vi "简易流程调试界面.vi"() -> ()   [LabVIEW 2016, in "斯坦道通用流路CODmn.lvlib"]
uses:
  <vilib>/Utility/miscctls.llb/LVPointTypeDef.ctl
  <vilib>/Plasmionique/MB Master/MB_Master/MB_Master.lvclass
panel:
  in  "调试控件":enum32{"填充流程", "清洗流程", "测试流程", "排空流程", "其他流程"}(tab)
  in  "填充简易流程":i32(listbox)
  in  "清洗简易流程":i32(listbox)
  in  "测试简易流程":i32(listbox)
  in  "排空简易流程":i32(listbox)
  in  "其他简易流程":i32(listbox)
  in  "停止":bool
  in  "单步测试":bool
  out "注射器温度":sgl
  out "消解温度":sgl
  out "ADC":sgl
  out "F3":sgl format="%#.6f"
  out "F2":sgl format="%#.6f"
  out "F1":sgl format="%#.6f"
  out "F0":sgl format="%#.6f"
  in  "启动":bool
  in  "参数下拉列表":u16(ring) items=["总磷"=1]
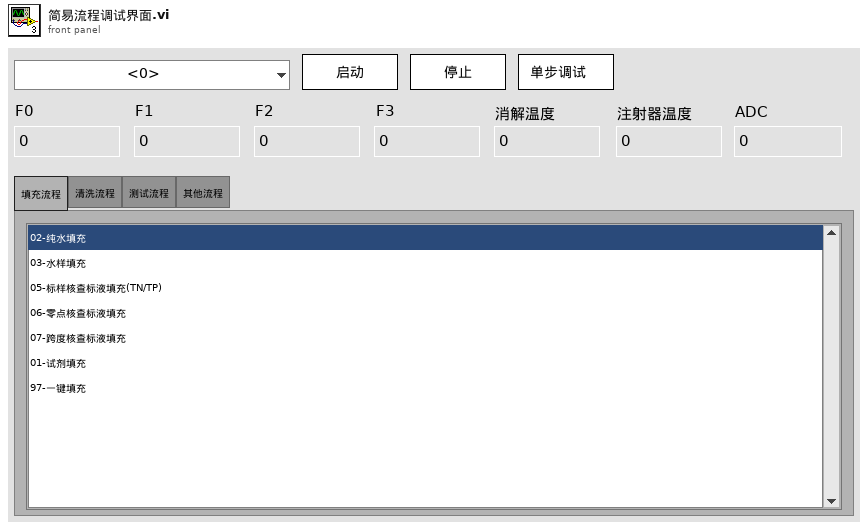
[diagram p1: front panel]
types:
  T1 = typedef "LVPointTypeDef.ctl" = cluster{"Horizontal":i16, "Vertical":i16}
  T2 = typedef "LVRectTypeDef.ctl" = cluster{"Left":i16, "Top":i16, "Right":i16, "Bottom":i16}
  T3 = typedef "LVStringsAndValuesArrayTypeDef_U16.ctl" = cluster{"String":string, "Value":u16}[]
  T4 = typedef "操作日志字段定义.ctl" = cluster{"时间":timestamp, "参数":string, "日志信息":string, "流程参数":string}
  T5 = enum16{"跨度核查", "水样测量", "零点核查", "标样核查", "加标回收", "快捷测试", "空白校准", "标样校准"}
  T6 = cluster{"系统时间":timestamp, "工作状态":u16, "测量模式":enum16{"待机", "连续模式", "周期模式", "定点模式", "受控模式", "手动模式"}, "告警代码":u16, "故障代码":u16, "日志代码":u16, "软件版本":u16, "F0":sgl, "F1":sgl, "F2":sgl, "F3":sgl, "T":sgl, "H":sgl, "id":u16, "flowid":u16, "量程":u16, "总磷控温温度1":sgl, "营养盐控温温度2":sgl, "ADC":sgl}
  T7 = enum32{"Bad", "Idle", "Run top level", "Running"}
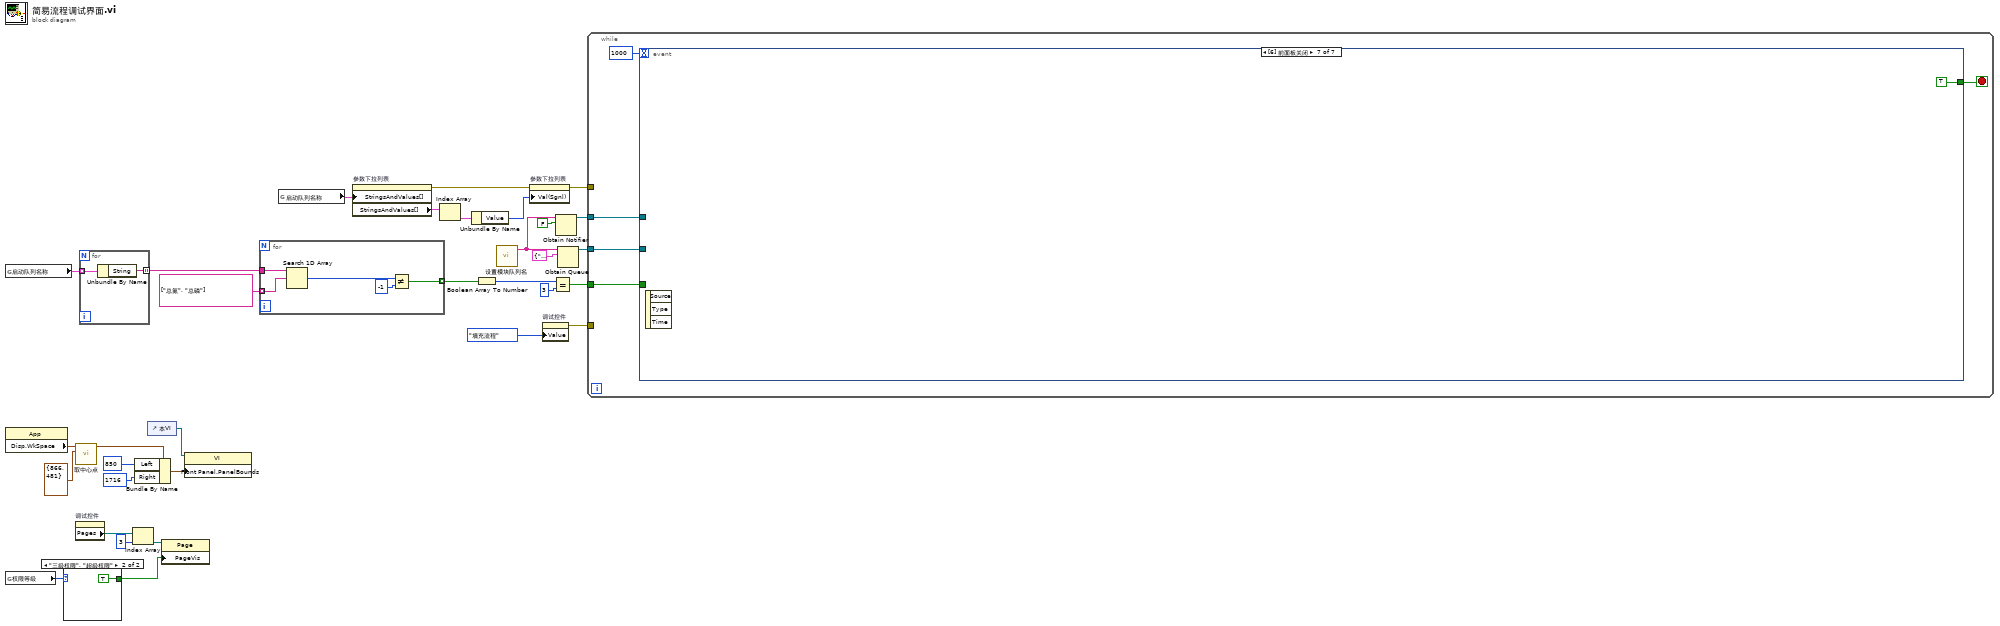
[diagram p0: block diagram]
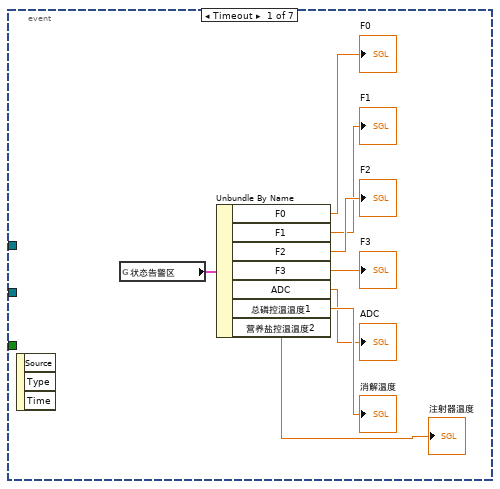
[diagram p3: hidden frame]
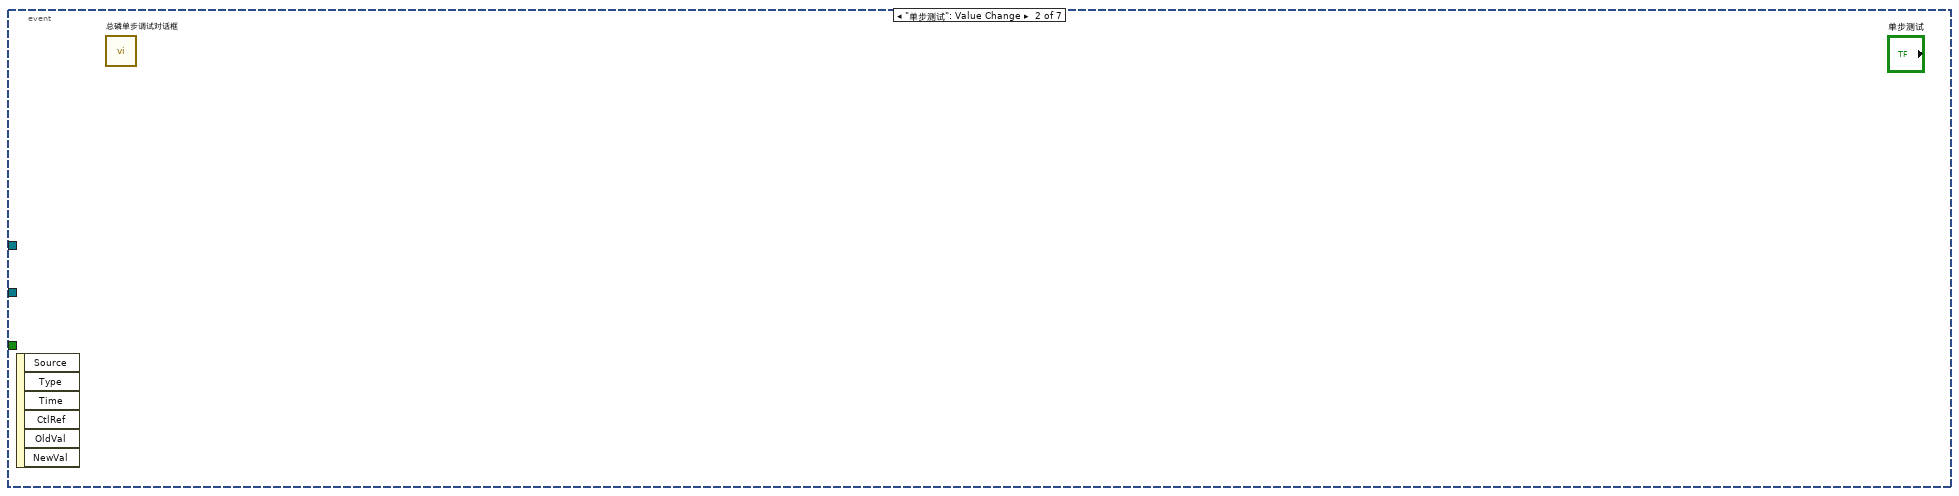
[diagram p4: hidden frame]
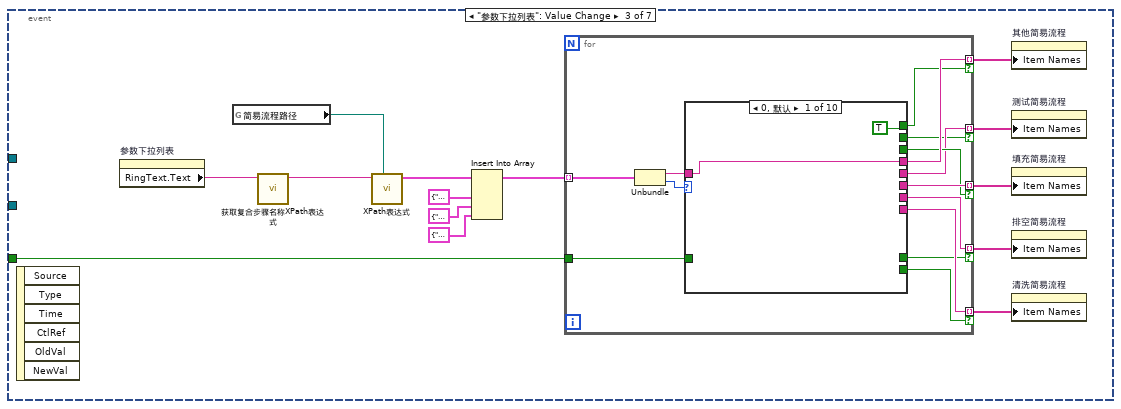
[diagram p5: hidden frame]
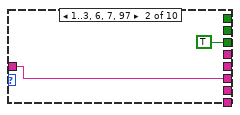
[diagram p6: hidden frame]
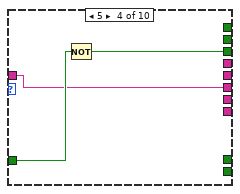
[diagram p8: hidden frame]
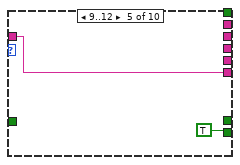
[diagram p9: hidden frame]
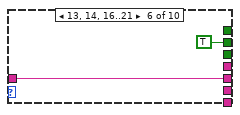
[diagram p10: hidden frame]
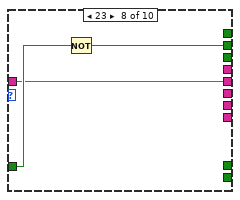
[diagram p12: hidden frame]
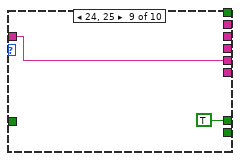
[diagram p13: hidden frame]
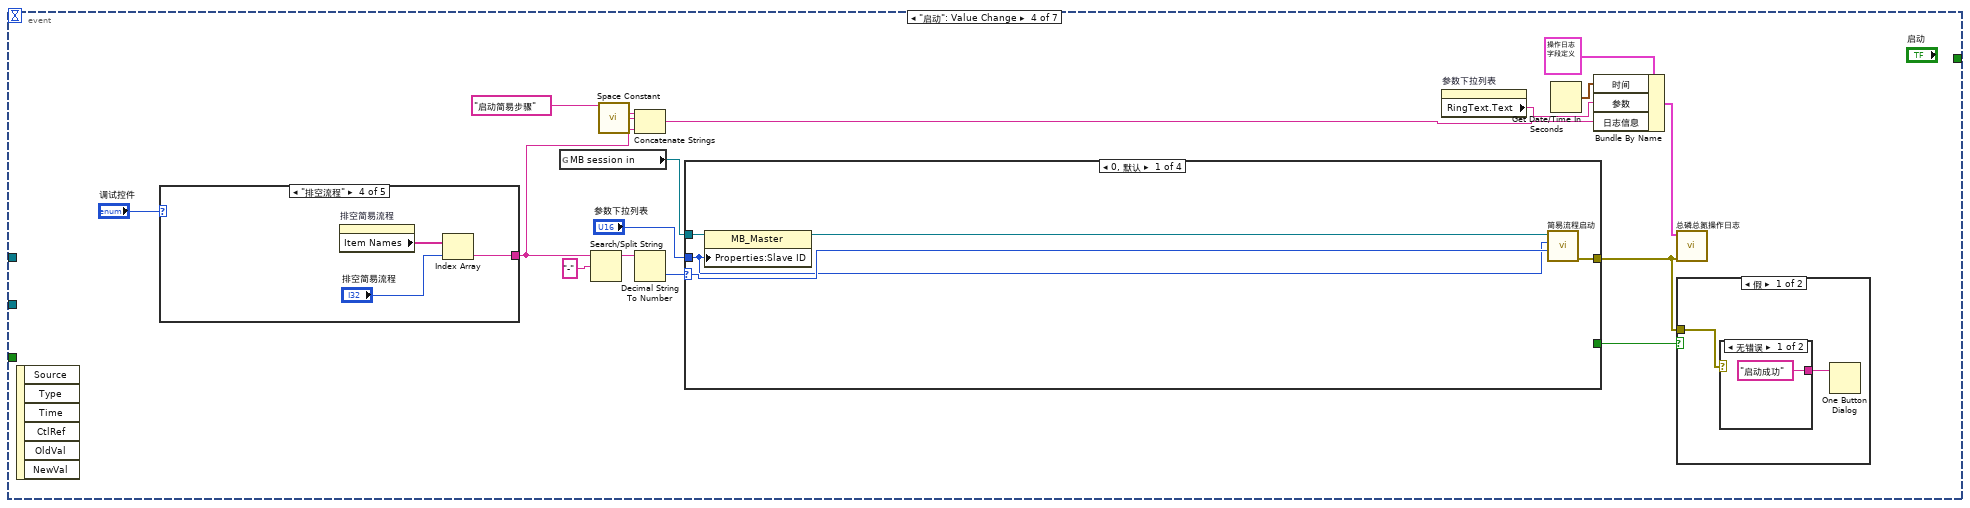
[diagram p15: hidden frame]
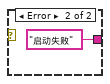
[diagram p16: hidden frame]
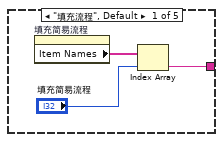
[diagram p18: hidden frame]
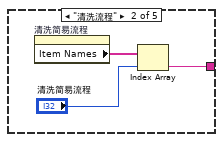
[diagram p19: hidden frame]
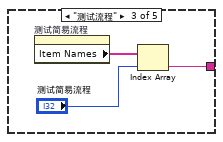
[diagram p20: hidden frame]
diagram:
  n1 = global read "model config var.vi" "启动队列名称"() -> (w3:cluster{"String":string, "Value":u16}[])
  n2 = property class="App"() -> ("Disp.WkSpace"=w13:T2)  [unwired: 2 in, 2 out]
  n3 = global read "VAR总磷总氮全局变量.vi" "权限等级"() -> (w19:enum16{"一级权限", "二级权限", "三级权限", "超级权限"})
  n4 = case shown="\"三级权限\", \"超级权限\"" w19 {
    tunnel: [_ TRUE ("选项卡可见")] -> w15
    frame "一级权限", Default {
    }
    frame "三级权限", "超级权限" {
    }
  }
  n5 = call "取中心点.vi"("前面板窗口:最小尺寸"=T1 {"Horizontal"=866, "Vertical"=481}, "显示:主工作区"=w13) -> ("前面板窗口:窗口边界"=w11:T2)  [unwired: 9 in]
  n6 = property on="调试控件" class="TabCtl (严格)"() -> ("Pages"=w18:refnum<vi>[])  [unwired: 2 in, 2 out]
  n7 = for {
    tunnel: w3 -> [w35] mode=indexing
    tunnel: [w34] -> w4 mode=indexing
    n8 = Unbundle By Name(w35) -> ("String"=w34:string)
  }
  n9 = Index Array(array=w18, index=3 ("索引")) -> (element=w16:refnum<vi>)
  n10 = Bundle By Name(cluster=w11, "Left"=i16 850, "Right"=i16 1716) -> (w10:T2)
  n11 = control-ref of="本VI"() -> (w14:refnum<vi>)
  n12 = property class="Page"(reference=w16, "PageVis"=w15) -> ()  [unwired: 1 in, 2 out]
  n13 = property class="VI"(reference=w14, "Front Panel.PanelBounds"=w10) -> ()  [unwired: 1 in, 2 out]
  n14 = for {
    tunnel: string[] ["总氮", "总磷"] -> [w39] mode=indexing
    tunnel: w4 -> [w40]
    tunnel: [w36] -> w5 mode=indexing
    n15 = Search 1D Array(1D array=w40, element=w39) -> (index of element=w38:i32)  [unwired: 1 in]
    n16 = Not Equal?(x=w38, y=-1) -> (x != y?=w36:bool)
  }
  n17 = global read "model config var.vi" "启动队列名称"() -> (w27:cluster{"String":string, "Value":u16}[])
  n18 = property on="参数下拉列表" class="Ring (严格)"("StringsAndValues[]"=w27) -> (error out=w28:errorcluster, "StringsAndValues[]"=w31:T3)  [unwired: 2 in, 1 out]
  n19 = Index Array(array=w31) -> (element=w30:cluster{"String":string, "Value":u16})  [unwired: 1 in]
  n20 = Unbundle By Name(w30) -> ("Value"=w29:u16)
  n21 = Boolean Array To Number(Boolean array=w5) -> (number=w6:u32)
  n22 = call "设置模块队列名.vi"() -> ("Msg"=w24:string)  [unwired: 5 in]
  n23 = property on="参数下拉列表" class="Ring (严格)"(error in=w28, "Val(Sgnl)"=w29) -> (error out=w32:errorcluster)  [unwired: 1 in, 1 out]
  n24 = property on="调试控件" class="TabCtl (严格)"("Value"=enum32{"填充流程", "清洗流程", "测试流程", "排空流程", "其他流程"}."填充流程" ("调试控件")) -> (error out=w20:errorcluster)  [unwired: 2 in, 1 out]
  n25 = Equal?(x=w6, y=u32 3) -> (x = y?=w1:bool)
  n26 = Obtain Notifier(name (unnamed)=w24, notification data type=FALSE) -> (notifier out=w23:refnum<notifier>)  [unwired: 2 in, 2 out]
  n27 = Obtain Queue(name (unnamed)=w24, element data type=cluster{"命令":string, "data":variant} {"命令"="", "data"=variant}) -> (queue out=w22:refnum<queue>)  [unwired: 3 in, 2 out]
  n28 = while {
    tunnel: w32 -> [_]
    tunnel: w23 -> [w43]
    tunnel: w22 -> [w42]
    tunnel: w20 -> [_]
    tunnel: w1 -> [w41]
    stop <- w45 stop-if-true
    n29 = event shown="[6] 前面板关闭" {
      selector: _ -> [_ _ _ _ _ _ _]
      dyn-events: _ -> [_ _ _ _ _ _ _]
      timeout: 1000 -> [_ _ _ _ _ _ _]
      tunnel: [_ _ _ _ _ _ TRUE] -> w45
      tunnel: w43 -> [_ _ _ _ _ w186 _]
      tunnel: w42 -> [_ _ _ _ _ w185 _]
      tunnel: w41 -> [_ _ w67 _ _ _ _]
      event Timeout {
        n30 = event-data() -> ()  [unwired: 1 in, 3 out]
        n31 = global read "VAR总磷总氮全局变量.vi" "状态告警区"() -> (w53:T6)
        n32 = Unbundle By Name(w53) -> ("F0"=→"F0":sgl, "F1"=→"F1":sgl, "F2"=→"F2":sgl, "F3"=→"F3":sgl, "ADC"=→"ADC":sgl, "总磷控温温度1"=→"消解温度":sgl, "营养盐控温温度2"=→"注射器温度":sgl)
      }
      event "单步测试": Value Change {
        n33 = event-data() -> ()  [unwired: 1 in, 6 out]
        n34 = call "总磷单步调试对话框.vi"() -> ()  [unwired: 12 in]
      }
      event "参数下拉列表": Value Change {
        n35 = event-data() -> ()  [unwired: 1 in, 6 out]
        n36 = property on="参数下拉列表" class="Ring (严格)"() -> ("RingText.Text"=w55:string)  [unwired: 2 in, 2 out]
        n37 = global read "总磷总氮断电保存全局变量.vi" "简易流程路径"() -> (w56:path)
        n38 = call "获取复合步骤名称XPath表达式.vi"("查询参数"=w55) -> ("Union"=w57:string)  [unwired: 10 in]
        n39 = call "XPath表达式.vi"("添加的路径"=w56, "XPath expression"=w57) -> ("数组"=w54:cluster{string, i32}[])  [unwired: 9 in]
        n40 = Insert Into Array(array=w54, new element #1=cluster{string, i32} {"97-一键填充", 97} ("新元素/子数组"), new element #2=cluster{string, i32} {"98-快捷测试（低量程）", 98} ("新元素/子数组"), new element #3=cluster{string, i32} {"99-快捷测试（高量程）", 99} ("新元素/子数组")) -> (w64:cluster{string, i32}[])  [unwired: 1 in]
        n41 = for {
          tunnel: w64 -> [w80] mode=indexing
          tunnel: [w79] -> w62 mode=indexing if=w78
          tunnel: [w77] -> w61 mode=indexing if=w76
          tunnel: [w75] -> w60 mode=indexing if=w74
          tunnel: [w73] -> w59 mode=indexing if=w72
          tunnel: [w71] -> w58 mode=indexing if=w70
          tunnel: w67 -> [w69]
          n42 = Unbundle(w80) -> (w68:string, w81:i32)
          n43 = case shown="0, 默认" w81 {
            tunnel: [w82 _ _ _ _ _ _ _ _ _] -> w79
            tunnel: [TRUE _ _ _ _ _ _ _ _ _] -> w78
            tunnel: [_ w84 w86 w88 _ _ _ _ _ _] -> w77
            tunnel: [_ TRUE w87 w89 _ _ _ _ _ _] -> w76
            tunnel: [_ _ _ _ w91 _ _ _ _ _] -> w75
            tunnel: [_ _ _ _ TRUE _ _ _ _ _] -> w74
            tunnel: [_ _ _ _ _ w93 w95 w97 _ _] -> w73
            tunnel: [_ _ _ _ _ TRUE w96 w98 _ _] -> w72
            tunnel: [_ _ _ _ _ _ _ _ w100 w102] -> w71
            tunnel: [_ _ _ _ _ _ _ _ TRUE _] -> w70
            tunnel: w69 -> [_ _ w87 w90 _ _ w96 w99 _ _]
            tunnel: w68 -> [w82 w84 w86 w88 w91 w93 w95 w97 w100 w102]
            frame 0, Default {
            }
            frame 1..3, 6, 7, 97 {
            }
            frame 4 {
            }
            frame 5 {
              n44 = Not(x=w90) -> (.not. x?=w89:bool)
            }
            frame 9..12 {
            }
            frame 13, 14, 16..21 {
            }
            frame 22 {
            }
            frame 23 {
              n45 = Not(x=w99) -> (.not. x?=w98:bool)
            }
            frame 24, 25 {
            }
            frame 8, 15 {
            }
          }
        }
        n46 = property on="其他简易流程" class="LstBox (严格)"("Item Names"=w62) -> ()  [unwired: 2 in, 2 out]
        n47 = property on="测试简易流程" class="LstBox (严格)"("Item Names"=w59) -> ()  [unwired: 2 in, 2 out]
        n48 = property on="填充简易流程" class="LstBox (严格)"("Item Names"=w61) -> ()  [unwired: 2 in, 2 out]
        n49 = property on="排空简易流程" class="LstBox (严格)"("Item Names"=w58) -> ()  [unwired: 2 in, 2 out]
        n50 = property on="清洗简易流程" class="LstBox (严格)"("Item Names"=w60) -> ()  [unwired: 2 in, 2 out]
      }
      event "启动": Value Change {
        n51 = event-data() -> ()  [unwired: 1 in, 6 out]
        n52 = case shown="\"排空流程\"" "调试控件" {
          tunnel: [w123 w126 w129 w132 w135] -> w104
          frame "填充流程", Default {
            n53 = property on="填充简易流程" class="LstBox (严格)"() -> ("Item Names"=w125:string[])  [unwired: 2 in, 2 out]
            n54 = Index Array(array=w125, index="填充简易流程") -> (element=w123:string)
          }
          frame "清洗流程" {
            n55 = property on="清洗简易流程" class="LstBox (严格)"() -> ("Item Names"=w128:string[])  [unwired: 2 in, 2 out]
            n56 = Index Array(array=w128, index="清洗简易流程") -> (element=w126:string)
          }
          frame "测试流程" {
            n57 = property on="测试简易流程" class="LstBox (严格)"() -> ("Item Names"=w131:string[])  [unwired: 2 in, 2 out]
            n58 = Index Array(array=w131, index="测试简易流程") -> (element=w129:string)
          }
          frame "排空流程" {
            n59 = property on="排空简易流程" class="LstBox (严格)"() -> ("Item Names"=w134:string[])  [unwired: 2 in, 2 out]
            n60 = Index Array(array=w134, index="排空简易流程") -> (element=w132:string)
          }
          frame "其他流程" {
            n61 = property on="其他简易流程" class="LstBox (严格)"() -> ("Item Names"=w137:string[])  [unwired: 2 in, 2 out]
            n62 = Index Array(array=w137, index="其他简易流程") -> (element=w135:string)
          }
        }
        n63 = global read "VAR总磷总氮全局变量.vi" "MB session in"() -> (w118:refnum<class "MB_Master.lvclass">)
        n64 = Search/Split String(string=w104, search string/char (-)="-" ("搜索字符串/字符(-)")) -> (substring before match=w114:string)  [unwired: 1 in, 2 out]
        n65 = call <vilib>:"Space Constant.vi"() -> ("String"=w103:string)
        n66 = Concatenate Strings("启动简易步骤" ("日志信息"), w103, w104) -> (w105:string)
        n67 = Decimal String To Number(string=w114) -> (number=w113:i32)  [unwired: 2 in, 1 out]
        n68 = case shown="0, 默认" w113 {
          selector: w113 -> [w140 w151 _ w172]
          tunnel: [w142 w152 _ w176] -> w106
          tunnel: w118 -> [w139 w150 _ w175]
          tunnel: "参数下拉列表" -> [w138 w149 w158 w174]
          tunnel: [_ w148 _ _] -> w112
          frame 0, Default {
            n69 = property class="MB_Master"(reference=w139, "Properties:Slave ID"=w138) -> (reference out=w141:refnum<class "MB_Master.lvclass">)  [unwired: 1 in, 1 out]
            n70 = call "简易流程启动.vi"("简易流程"=w140, "参数Id"=w138, "MB session in"=w141) -> ("error out"=w142:errorcluster)  [unwired: 7 in, 1 out]
          }
          frame 24 {
            n71 = call "警示对话框.vi"("副标题颜色"=u32 0, "主标题颜色"=u32 16711680, "副标题"="请确认所有试剂均已拆除，除纯水管外所有管路接入废液桶（瓶）！" ("消息"), "主标题"="警告！！！" ("消息")) -> ("check"=w143:bool)  [unwired: 7 in]
            n72 = Not(x=w143) -> (.not. x?=w148:bool)
            n73 = case shown="真" w143 {
              tunnel: [_ w157] -> w152
              tunnel: w151 -> [_ w155]
              tunnel: w150 -> [_ w154]
              tunnel: w149 -> [_ w153]
              frame False {
              }
              frame True {
                n74 = property class="MB_Master"(reference=w154, "Properties:Slave ID"=w153) -> (reference out=w156:refnum<class "MB_Master.lvclass">)  [unwired: 1 in, 1 out]
                n75 = call "简易流程启动.vi"("简易流程"=w155, "参数Id"=w153, "MB session in"=w156) -> ("error out"=w157:errorcluster)  [unwired: 7 in, 1 out]
              }
            }
          }
          frame 97 {
            n76 = vi-ref "一键清洗流程.vi"() -> (w159:refnum<vi>)
            n77 = property class="VI"(reference=w159) -> ("Name"=w160:string, "Exec.State"=w161:T7)  [unwired: 1 in, 2 out]
            n78 = case shown="\"Idle\"" w161 {
              tunnel: w160 -> [_ w170]
              tunnel: w158 -> [_ w163]
              frame "Bad", Default {
              }
              frame "Idle" {
                n79 = property on="填充简易流程" class="LstBox (严格)"() -> ("Item Names"=w162:string[])  [unwired: 2 in, 2 out]
                n80 = Open VI Reference(type specifier VI Refnum (for type only)=refnum<vi> refnum, vi path=w170, options=128 ("选项")) -> (vi reference=w167:refnum<vi>, error out=w165:errorcluster)  [unwired: 3 in]
                n81 = call-by-ref "开始异步调用"(reference=w167, error in=w165, "项名"=w162, "参数下拉列表"=w163) -> (reference out=w166:refnum<vi>, error out=w164:errorcluster)  [unwired: 10 in]
                n82 = Close Reference(reference=w166, error in (no error)=w164) -> ()  [unwired: 1 out]
              }
            }
          }
          frame 98, 99 {
            n83 = case shown="98, 默认" w172 {
              tunnel: [enum16{"低量程", "高量程"}."低量程" ("量程下拉列表") enum16{"低量程", "高量程"}."高量程" ("量程下拉列表")] -> w171
              frame 98, Default {
              }
              frame 99 {
              }
            }
            n84 = call "非国标启动命令.vi"("参数下拉列表"=w174, "量程下拉列表"=w171, "测量模式"=T5."快捷测试", "MB session in"=w175) -> ("error out"=w176:errorcluster)  [unwired: 6 in, 1 out]
          }
        }
        n85 = property on="参数下拉列表" class="Ring (严格)"() -> ("RingText.Text"=w108:string)  [unwired: 2 in, 2 out]
        n86 = Get Date/Time In Seconds() -> (seconds since 1Jan1904=w109:timestamp)
        n87 = Bundle By Name(cluster=T4 {"时间"=timestamp(0 s since 1904-01-01), "参数"="", "日志信息"="", "流程参数"=""} ("data in"), "时间"=w109, "参数"=w108, "日志信息"=w105) -> (w110:T4)
        n88 = call "总磷总氮操作日志.vi"("错误输入（无错误）"=w106, "data in"=w110) -> ()  [unwired: 9 in, 1 out]
        n89 = case shown="假" w112 {
          tunnel: w106 -> [w120 _]
          frame False {
            n90 = case shown="无错误" w120 {
              tunnel: ["启动成功" "启动失败"] -> w119
              frame No Error {
              }
              frame Error {
              }
            }
            n91 = One Button Dialog(message=w119) -> ()  [unwired: 1 in, 1 out]
          }
          frame True {
          }
        }
      }
      event "排空简易流程": Mouse Down {
        n92 = event-data() -> ()  [unwired: 1 in, 6 out]
      }
      event "停止": Value Change {
        n93 = event-data() -> ()  [unwired: 1 in, 6 out]
        n94 = Send Notification(notification=TRUE ("通知"), notifier=w186) -> ()  [unwired: 1 in, 2 out]
        n95 = Enqueue Element(queue=w185, element=cluster{"命令":string, "data":variant} {"命令"="启动", "data"=variant(cluster{"站号":u16, "控制命令输出":u16[]} {"站号"=1, "控制命令输出"=[2816]})} ("元素")) -> (queue out=w188:refnum<queue>)  [unwired: 2 in, 2 out]
        n96 = property on="参数下拉列表" class="Ring (严格)"() -> ("RingText.Text"=w179:string)  [unwired: 2 in, 2 out]
        n97 = Get Date/Time In Seconds() -> (seconds since 1Jan1904=w182:timestamp)
        n98 = Enqueue Element(queue=w188, element=cluster{"命令":string, "data":variant} {"命令"="启动", "data"=variant(cluster{"站号":u16, "控制命令输出":u16[]} {"站号"=2, "控制命令输出"=[2816]})} ("元素")) -> (error out=w180:errorcluster)  [unwired: 2 in, 2 out]
        n99 = Bundle By Name(cluster=T4 {"时间"=timestamp(0 s since 1904-01-01), "参数"="", "日志信息"="", "流程参数"=""} ("data in"), "时间"=w182, "参数"=w179, "日志信息"="手动停止") -> (w183:T4)
        n100 = call "总磷总氮操作日志.vi"("错误输入（无错误）"=w180, "data in"=w183) -> ()  [unwired: 9 in, 1 out]
      }
      event Panel Close {
        n101 = event-data() -> ()  [unwired: 1 in, 3 out]
      }
    }
  }
